vi "Save_Converted.vi"(6 "Top level VI Name":string, 8 "Vi's already saved in":string[](array[string]), 9 "Saved Vis paths in":string[](array[string]), 10 "VI to save":string, 11 "vi reference":refnum<vi>) -> (0 "Vi's already saved out":string[](array[string]), 1 "Error IO":errorcluster, 2 "vi references to save":refnum<vi>[](array[refnum]), 3 "Vi's that need saving":string[](array[string]), 4 "Saved Vis paths Out":string[](array[string]))   [LabVIEW 2020]
panel:
  out "VIType":T1(ring)
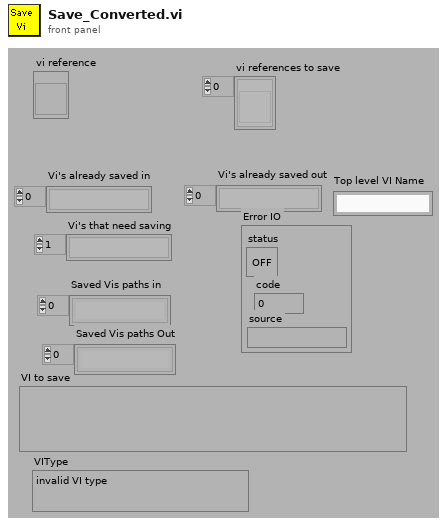
[diagram p1: front panel]
types:
  T1 = enum32{"invalid VI type", "Standard VI", "Control VI", "Global VI"}
  T2 = enum32{"invalid VI type", "Standard VI", "Control VI", "Global VI", "Polymorphic VI", "Configuration VI", "SubSystem", "Facade VI", "Method VI", "Statechart Diagram VI"}
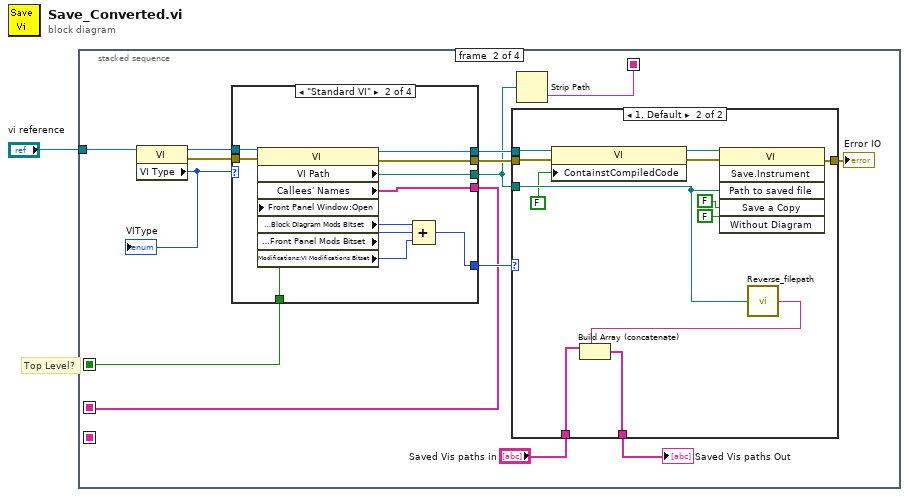
[diagram p0: block diagram]
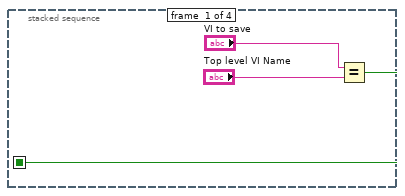
[diagram p2: hidden frame]
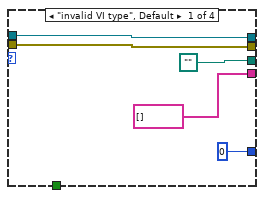
[diagram p3: hidden frame]
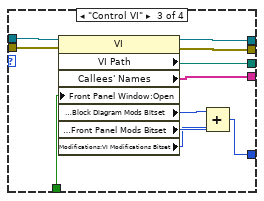
[diagram p4: hidden frame]
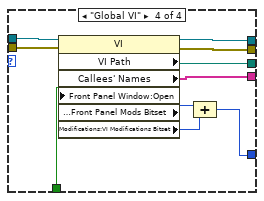
[diagram p5: hidden frame]
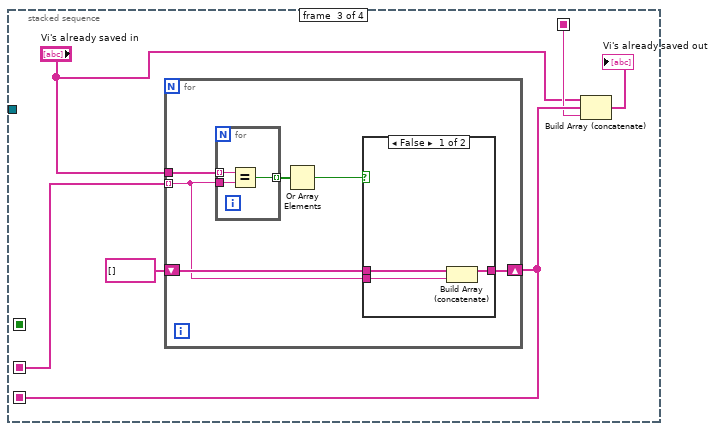
[diagram p7: hidden frame]
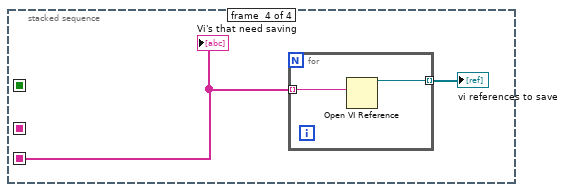
[diagram p9: hidden frame]
diagram:
  # "Top Level?"
  n1 = stacked-sequence {
    seq-local: [_ w12 _ _] -> [_ _ w75 _]
    seq-local: [_ _ w73 _] -> [_ _ _ w90]
    seq-local: [_ w11 _ _] -> [_ _ w71 _]
    seq-local: [w2 _ _ _] -> [_ w5 _ _]
    tunnel: "vi reference" -> [_ w7 _ _]
    frame #0 {
      n2 = Equal?(x="VI to save", y="Top level VI Name") -> (x = y?=w2:bool)
    }
    frame #1 {
      n3 = property class="VI"(reference=w7) -> (reference out=w14:refnum<vi>, error out=w13:errorcluster, "VI Type"=w15:T2)  [unwired: 1 in]
      "VIType" <- w15
      n4 = case shown="\"Standard VI\"" w15 {
        tunnel: [string[] [] ("Callees") w34 w45 w55] -> w12
        tunnel: [path "" ("Path") w33 w44 w54] -> w6
        tunnel: [w21 w32 w43 w53] -> w18
        tunnel: [w22 w31 w42 w52] -> w17
        tunnel: w14 -> [w21 w30 w41 w51]
        tunnel: [u32 0 w24 w37 w47] -> w16
        tunnel: w13 -> [w22 w29 w40 w50]
        tunnel: w5 -> [_ w28 w36 w46]
        frame "invalid VI type", Default {
        }
        frame "Standard VI" {
          n5 = property class="VI"(reference=w30, error in=w29, "Front Panel Window:Open"=w28) -> (reference out=w32:refnum<vi>, error out=w31:errorcluster, "VI Path"=w33:path, "Callees' Names"=w34:string[], "Modifications:Block Diagram Mods Bitset"=w27:u32, "Modifications:Front Panel Mods Bitset"=w26:u32, "Modifications:VI Modifications Bitset"=w25:u32)
          n6 = Compound Arithmetic op=ADD(w27, w26, w25) -> (w24:u32)
        }
        frame "Control VI" {
          n7 = property class="VI"(reference=w41, error in=w40, "Front Panel Window:Open"=w36) -> (reference out=w43:refnum<vi>, error out=w42:errorcluster, "VI Path"=w44:path, "Callees' Names"=w45:string[], "Modifications:Block Diagram Mods Bitset"=w39:u32, "Modifications:Front Panel Mods Bitset"=w38:u32, "Modifications:VI Modifications Bitset"=w35:u32)
          n8 = Compound Arithmetic op=ADD(w39, w38, w35) -> (w37:u32)
        }
        frame "Global VI" {
          n9 = property class="VI"(reference=w51, error in=w50, "Front Panel Window:Open"=w46) -> (reference out=w53:refnum<vi>, error out=w52:errorcluster, "VI Path"=w54:path, "Callees' Names"=w55:string[], "Modifications:Front Panel Mods Bitset"=w49:u32, "Modifications:VI Modifications Bitset"=w48:u32)
          n10 = Compound Arithmetic op=ADD(w49, w48) -> (w47:u32)
        }
      }
      n11 = case shown="1, Default" w16 {
        tunnel: w6 -> [_ w64]
        tunnel: w18 -> [_ w62]
        tunnel: w17 -> [w57 w61]
        tunnel: [w57 w67] -> w8
        tunnel: [w56 w65] -> w10
        tunnel: "Saved Vis paths in" -> [w56 w66]
        frame 0 {
        }
        frame 1, Default {
          n12 = property class="VI"(reference=w62, error in=w61, "ContainstCompiledCode"=FALSE ("Contains Compiled Code")) -> (reference out=w60:refnum<vi>, error out=w59:errorcluster)
          n13 = invoke class="VI" method="Save.Instrument"(reference=w60, error in=w59, "Path to saved file"=w64, "Save a Copy"=FALSE, "Without Diagram"=FALSE) -> (error out=w67:errorcluster)  [unwired: 1 in, 5 out]
          n14 = call "Reverse_filepath.vi"("Filename"=w64) -> ("Reversed Filepath"=w63:string)
          n15 = Build Array (concatenate)(w66, w63) -> (w65:string[])
        }
      }
      "Error IO" <- w8
      "Saved Vis paths Out" <- w10
      n16 = Strip Path(path=w6) -> (name=w11:string)  [unwired: 1 out]
    }
    frame #2 {
      n17 = for {
        tunnel: w75 -> [w79] mode=indexing
        tunnel: "Vi's already saved in" -> [w78]
        shift-right: [w80] -> w73
        shift-left: string[] [] -> [w81]
        n18 = for {
          tunnel: w79 -> [w84]
          tunnel: w78 -> [w83] mode=indexing
          tunnel: [w82] -> w77 mode=indexing
          n19 = Equal?(x=w83, y=w84) -> (x = y?=w82:bool)
        }
        n20 = Or Array Elements(Boolean array=w77) -> (logical OR=w76:bool)
        n21 = case shown="False" w76 {
          tunnel: w79 -> [w87 _]
          tunnel: w81 -> [w86 w88]
          tunnel: [w85 w88] -> w80
          frame False {
            n22 = Build Array (concatenate)(w86, w87) -> (w85:string[])
          }
          frame True {
          }
        }
      }
      n23 = Build Array (concatenate)("Vi's already saved in", w73, w71) -> (→"Vi's already saved out":string[])
    }
    frame #3 {
      n24 = for {
        tunnel: w90 -> [w92] mode=indexing
        tunnel: [w91] -> w89 mode=indexing
        n25 = Open VI Reference(vi path=w92) -> (vi reference=w91:refnum<vi>)  [unwired: 1 in, 5 out]
      }
      "vi references to save" <- w89
      "Vi's that need saving" <- w90
    }
  }
